vi "SubVI_Img2Mat_001.vi"(0 "Path":path) -> (1 "Picture":picture, 2 "1-bit pixmap":bool[][](array[boolean]))   [LabVIEW 2018]
uses:
  <vilib>/picture/picture.llb/Draw 1-Bit Pixmap.vi
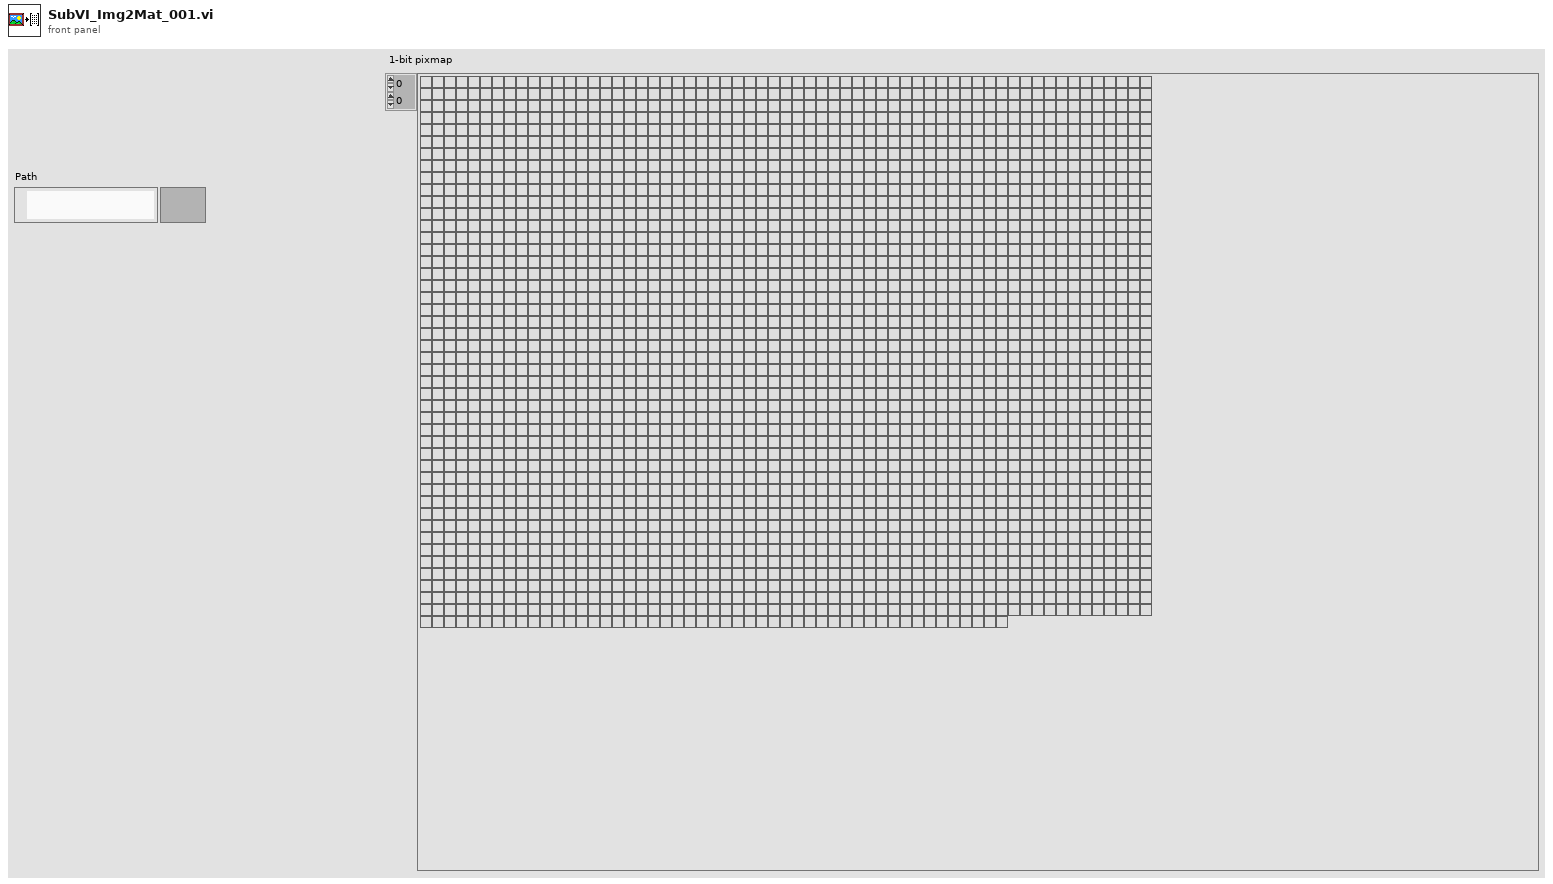
[diagram p1: front panel]
types:
  T1 = typedef "imagedata.ctl" = cluster{"image type":i32, "image depth":i32, "image":u8[], "mask":u8[], "colors":u32[], "Rectangle":cluster{"left":i16, "top":i16, "right":i16, "bottom":i16}}
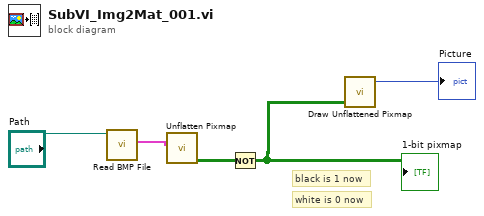
[diagram p0: block diagram]
diagram:
  # "white is 0 now"
  # "black is 1 now"
  n1 = call <vilib>:"Read BMP File.vi"("path to BMP file"="Path") -> ("image data"=w4:T1)  [unwired: 8 in, 2 out]
  n2 = call <vilib>:"Unflatten Pixmap.vi"("image data"=w4) -> ("1-bit pixmap"=w2:bool[][])  [unwired: 4 in, 6 out]
  n3 = Not(x=w2) -> (.not. x?=w1:bool[][])
  "1-bit pixmap" <- w1
  n4 = call-poly <vilib>:"Draw Unflattened Pixmap.vi"("data"=w1) -> ("new picture"=→"Picture":picture)  [unwired: 8 in]
